vi "Error.vi"(8 "error in (no error)":errorcluster caption="错误输入（无错误）", 11 "VISA资源名称":refnum<visa-resource-name>) -> (0 "错误输出":errorcluster, 1 "全部错误消息":string, 2 "错误代码数组":i32[](array[numeric]), 3 "VISA引用句柄输出":refnum<visa-resource-name>)   [LabVIEW 2018]
doc: "错误处理"
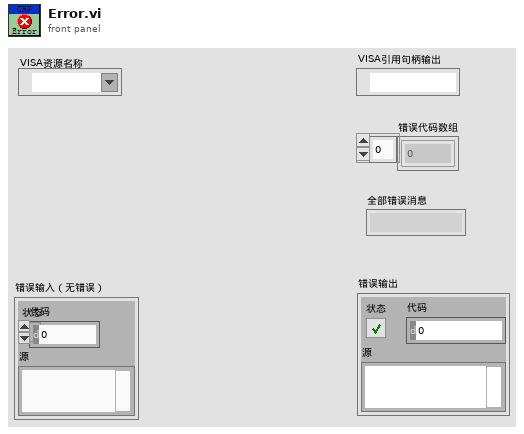
[diagram p1: front panel]
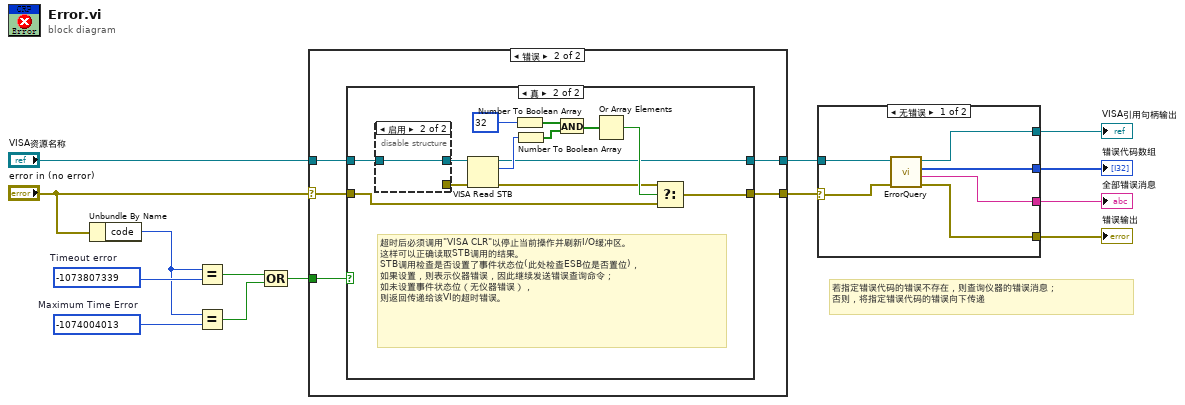
[diagram p0: block diagram]
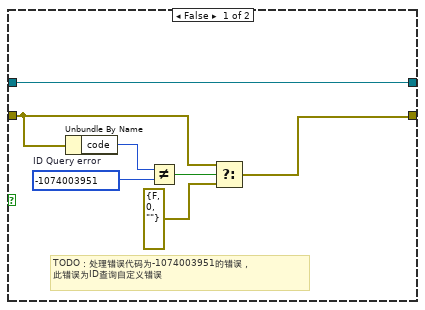
[diagram p4: hidden frame]
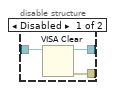
[diagram p5: hidden frame]
diagram:
  w13 = -1074004013  # Maximum Time Error
  w14 = -1073807339  # Timeout error
  # "若指定错误代码的错误不存在，则查询仪器的错误消息；\n否则，将指定错误代码的错误向下传递"
  n1 = Unbundle By Name("error in (no error)") -> ("code"=w12:i32)
  n2 = Equal?(x=w12, y=w14) -> (x = y?=w10:bool)
  n3 = Equal?(x=w12, y=w13) -> (x = y?=w9:bool)
  n4 = Compound Arithmetic op=OR ("复合运算")(w10, w9) -> (w8:bool)
  n5 = case shown="错误" "error in (no error)" {
    selector: "error in (no error)" -> [w15 w19]
    tunnel: w8 -> [_ w21]
    tunnel: "VISA资源名称" -> [w16 w20]
    tunnel: [w15 w18] -> w6
    tunnel: [w16 w17] -> w5
    frame No Error {
    }
    frame Error {
      n6 = case shown="真" w21 {
        tunnel: w20 -> [w28 w41]
        tunnel: w19 -> [w24 w32]
        tunnel: [w28 w30] -> w17
        tunnel: [w22 w29] -> w18
        frame False {
          w26 = -1074003951  # ID Query error
          # "TODO：处理错误代码为-1074003951的错误，\n此错误为ID查询自定义错误"
          n7 = Unbundle By Name(w24) -> ("code"=w27:i32)
          n8 = Not Equal?(x=w27, y=w26) -> (x != y?=w25:bool)
          n9 = Select(t=w24, s=w25, f=errorcluster {"status"=FALSE, "code"=0, "source"=""}) -> (s? t:f=w22:errorcluster)
        }
        frame True {
          # "超时后必须调用\"VISA CLR\"以停止当前操作并刷新I/O缓冲区。\n这样可以正确读取STB调用的结果。 \nSTB调用检查是否设置了事件状态位(此处检查ESB位是否置位)，\n如果设置，则表示仪器错误，因此继续发送错误查询命令；\n如未设置事件状态位（无仪器错误），\n则返回传递给该VI的超时错误。"
          n10 = disable-structure shown="启用" {
            disable-tunnel: w41 -> [w44 w45]
            disable-tunnel: [w43 w45] -> w40
            disable-tunnel: [w42 _] -> w39
            frame Disabled {
              n11 = VISA Clear(VISA resource name=w44) -> (VISA resource name out=w43:refnum<visa-resource-name>, error out=w42:errorcluster)  [unwired: 1 in]
            }
            frame Enabled {
            }
          }
          n12 = VISA Read STB(8:w39, 11:w40) -> (0:w31:errorcluster, 2:w37:u16, 3:w30:refnum<visa-resource-name>)
          n13 = Number To Boolean Array(number=u16 32) -> (Boolean array=w36:bool[])
          n14 = Number To Boolean Array(number=w37) -> (Boolean array=w35:bool[])
          n15 = And(x=w36, y=w35) -> (x .and. y?=w34:bool[])
          n16 = Or Array Elements(Boolean array=w34) -> (logical OR=w33:bool)
          n17 = Select(t=w31, s=w33, f=w32) -> (s? t:f=w29:errorcluster)
        }
      }
    }
  }
  n18 = case shown="无错误" w6 {
    selector: w6 -> [w50 w52]
    tunnel: w5 -> [w51 w53]
    tunnel: [w49 w53] -> w4
    tunnel: [w48 _] -> w3
    tunnel: [w47 _] -> w1
    tunnel: [w46 w52] -> w2
    frame No Error {
      n19 = call "ErrorQuery.vi"("错误输入（无错误）"=w50, "VISA引用句柄输入"=w51) -> ("错误输出"=w46:errorcluster, "全部错误消息"=w47:string, "错误代码数组"=w48:i32[], "VISA引用句柄输出"=w49:refnum<visa-resource-name>)  [unwired: 6 in]
    }
    frame Error {
    }
  }
  "VISA引用句柄输出" <- w4
  "错误代码数组" <- w3
  "错误输出" <- w2
  "全部错误消息" <- w1
